vi "main.vi"() -> ()   [LabVIEW 2018]
uses:
  Classes/Main/Status STYP.ctl
  Classes/Video Processor/Video Processor.lvclass
  C:/Users/aaron.jencks/Documents/GitHub/emerson_seed_object_detection/LabVIEW/Projects/Paul's Video Viewer/Classes/Video File/Video File.lvclass
  <vilib>/vision/Image Controls.llb/IMAQ Image.ctl
  <userlib>/Jet Engineering/JET_QSM/Code/Private/JET_QSM_InvalidOption STYP.ctl
  Classes/Video File/Video File.lvclass/Video File.ctl
  <userlib>/Jet Engineering/JET_QSM/Code/Private/JET_QSM - Add State [String API].vi
  3189c987-d43a-4d5a-91ed-d680ee457747.vi
  bcec0ad0-729b-4a4f-bcea-59fd1ae3eb4f.vi
  Classes/Video File/Read Number of Frames.vi
  Classes/Video File/Read Frame Number.vi
  Classes/Standard RMS/Standard RMS.lvclass
  C:/Users/aaron.jencks/Documents/GitHub/emerson_seed_object_detection/LabVIEW/Projects/Paul's Video Viewer/Classes/Standard Averager/Standard Averager.lvclass
  <vilib>/Utility/error.llb/Trim Whitespace.vi
  <vilib>/Utility/error.llb/Error Cluster From Error Code.vi
  Classes/Standard Averager/Standard Averager.lvclass
panel:
  out "Frame Number B":u32
  out "Frame Number A":u32
  in  "Depth Value Boundaries":cluster{dbl, dbl}(slide)={0.0, 7.2727272727272725} scale=0.0..5.0
  in  "Position Boundaries B":cluster{u32, u32}(slide)={0, 99} caption="Playback Boundaries" scale=0.0..298.0
  in  "Position Boundaries A":cluster{u32, u32}(slide)={0, 44} caption="Playback Boundaries" scale=0.0..249.0
  in  "Depth Scale B":dbl caption="Depth Scale"
  in  "Depth Scale A":dbl caption="Depth Scale"
  in  "Averaging Type":enum32{"Normal Average", "RMS"}(radio)
  out "Video B Info":cluster{"Roughness":dbl, "Average Depth":dbl} {"Roughness" format="%#.3g"; "Average Depth" format="%#.3g"}
  out "Video A Info":cluster{"Roughness":dbl, "Average Depth":dbl} {"Roughness" format="%#.3g"; "Average Depth" format="%#.3g"}
  in  "Restart":bool
  in  "stop":bool
  in  "Depth History Length (-1: Infinite)":i32=10
  out "Playback Position":dbl(slide) scale=0.0..100.0
  in  "Pause":bool
  in  "Play":bool
  in  "Video Path B":path
  in  "Video Path A":path
  in  "FPS":dbl(slide) scale=1.0..15.0
  out "Recent states before Error (with tick counts) 2":string="0.167 sec ago: VI Initialize\n0.167 sec ago: Window Open\n0.110 sec ago: Control Update\n0.110 sec ago: Indicator Update\n0.000 sec ago: Error Handler\r\n"
  out "error out":errorcluster
  out "Video Frame B":T1(plugin-control)
  out "Video Frame A":T1(plugin-control)
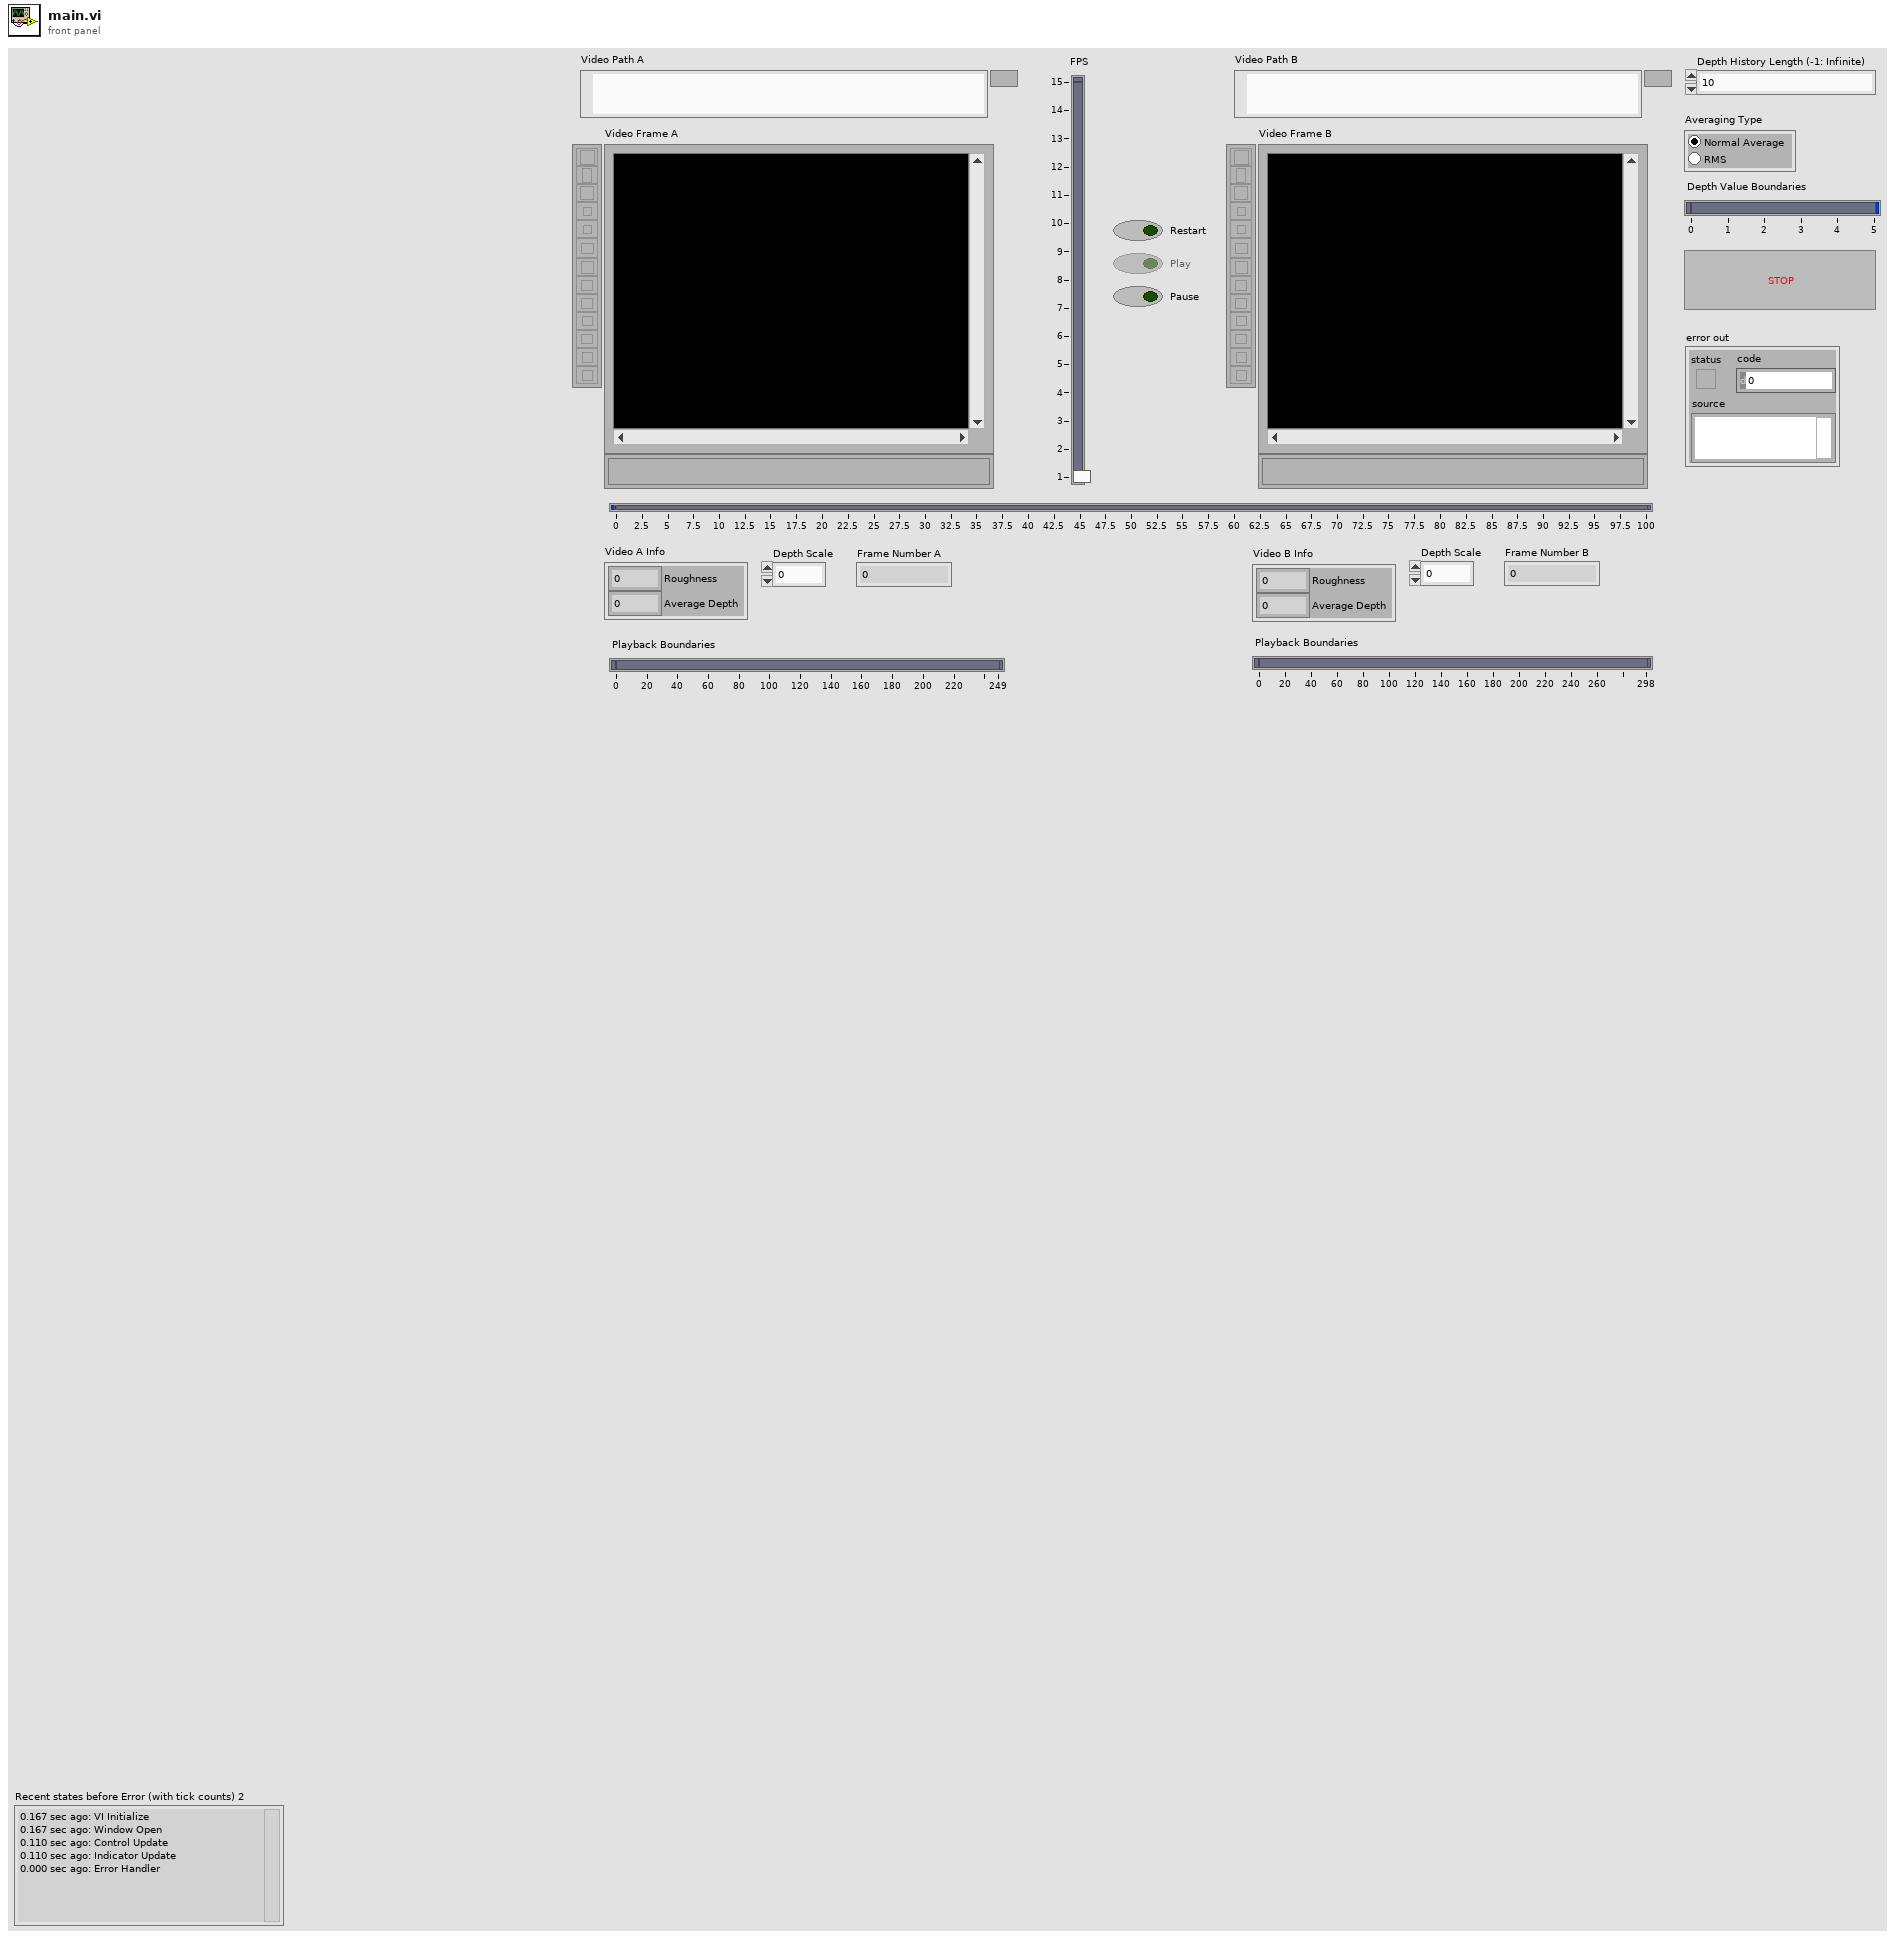
[diagram p1: front panel]
types:
  T1 = typedef "IMAQ Image.ctl" = refnum<image>
  T2 = typedef "Status STYP.ctl" = cluster{"VI":cluster{"error":errorcluster, "isExiting?":bool}, "UserLoggedIn?":bool, "Processors":cluster{"Video A":refnum<class "Video Processor.lvclass">, "Video B":refnum<class "Video Processor.lvclass">, "Averaging Type":enum32{"Normal Average", "RMS"}}, "Playback":cluster{"FPS":dbl, "Playing?":bool, "Playable?":bool, "Image A":T1, "Image B":T1}}
  T3 = typedef "JET_QSM_InvalidOption STYP.ctl" = enum16{"Ignore", "Dialog", "Error"}
  T4 = typedef "JET_QSM_Refnum STYP.ctl" = cluster{"state":cluster{"queue":refnum<queue>, "idle":string, "error":string, "STOP":string}, "debug":cluster{"enabled?":bool, "queue":refnum<queue>}, "Invalid.option":T3, "QSM.Name":string}
  T5 = enum32{"invalid app kind", "Development System", "Run Time System", "Student Edition", "Embedded LabVIEW", "Evaluation", "Custom"}
  T6 = typedef "Image Type" = u32
  T7 = cluster{"Global Rectangle":i32[], "Contours":cluster{"Contour Type":u32, "ROI Type":u32, "Points":i32[]}[]}
  T8 = typedef "JET_QSM_Element STYP.ctl" = cluster{"state":string, "data":variant, "comment":string}
  T9 = cluster{"Number of Frames":u32, "Accessors:Number of Frames":u32}
  T10 = cluster{"Accessors:History Standard Deviation":dbl, "Accessors:History Average":dbl}
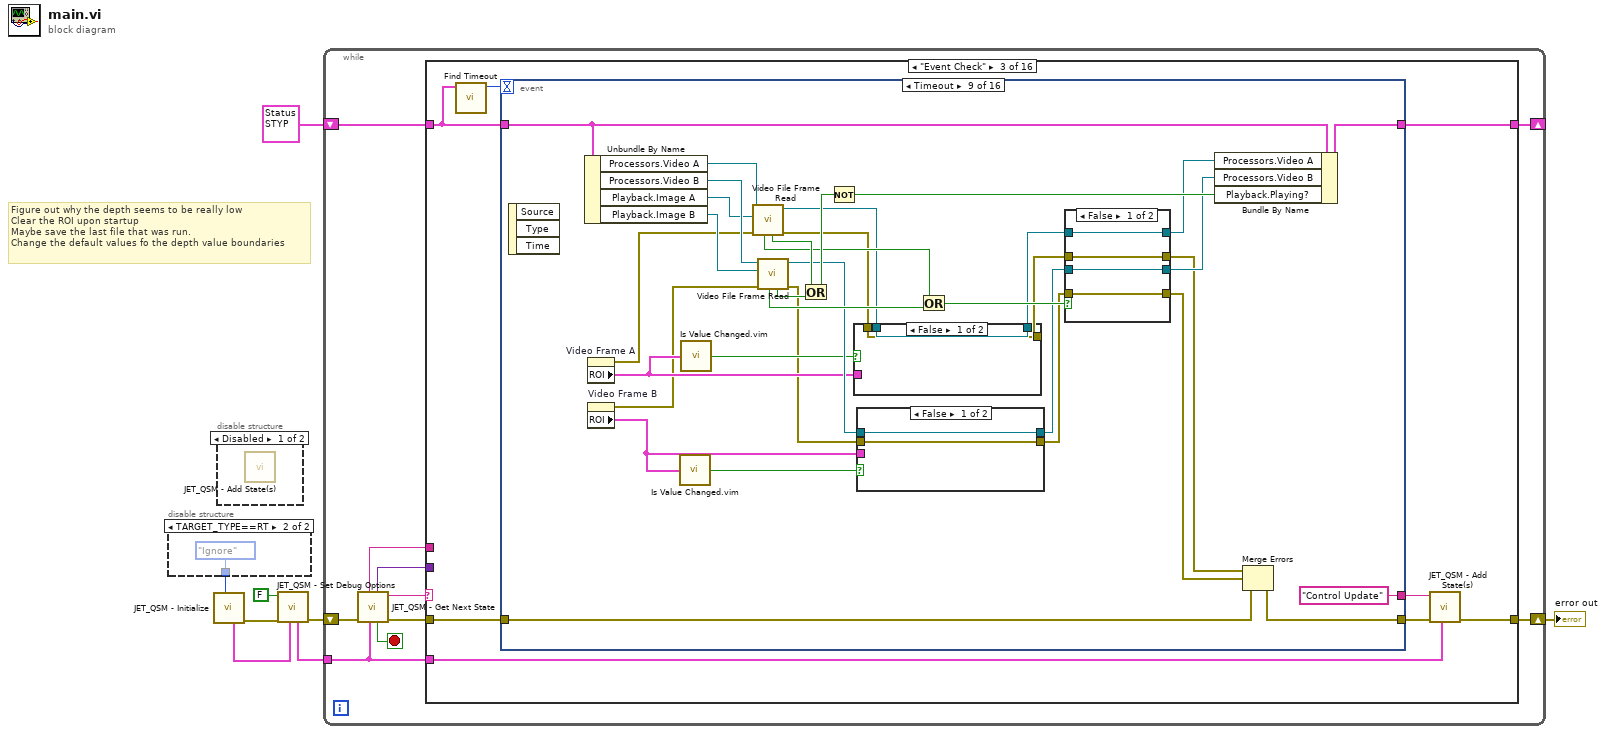
[diagram p0: block diagram]
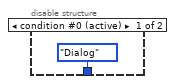
[diagram p2: hidden frame]
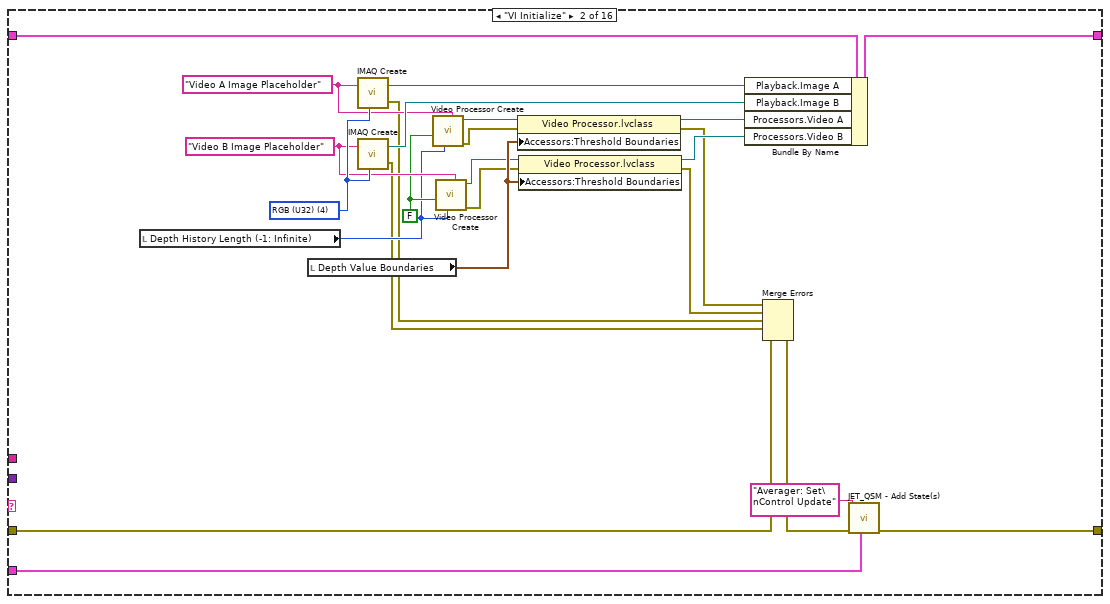
[diagram p5: hidden frame]
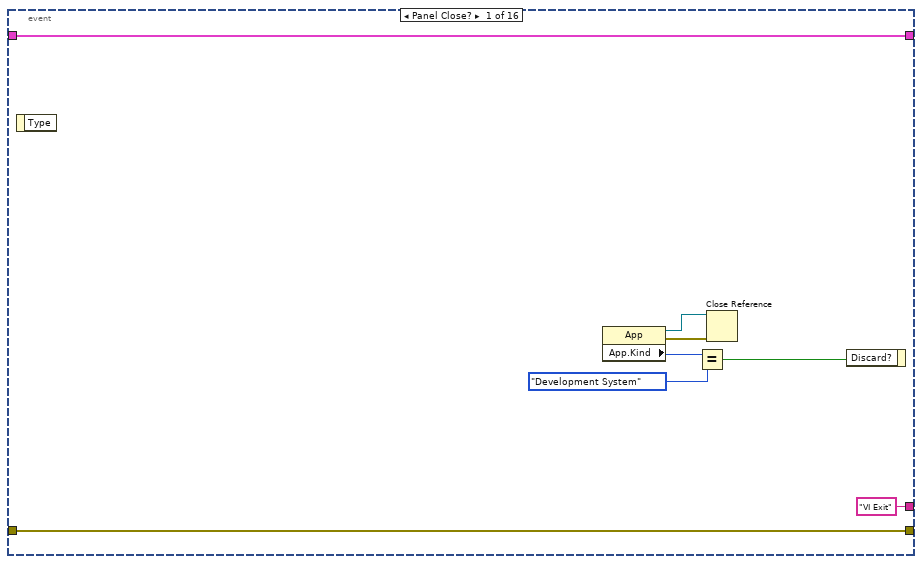
[diagram p6: hidden frame]
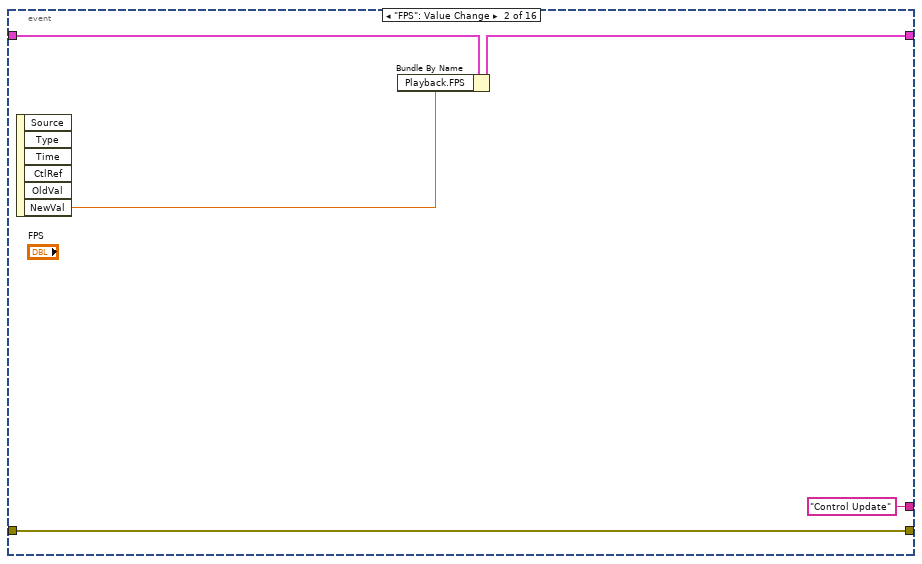
[diagram p7: hidden frame]
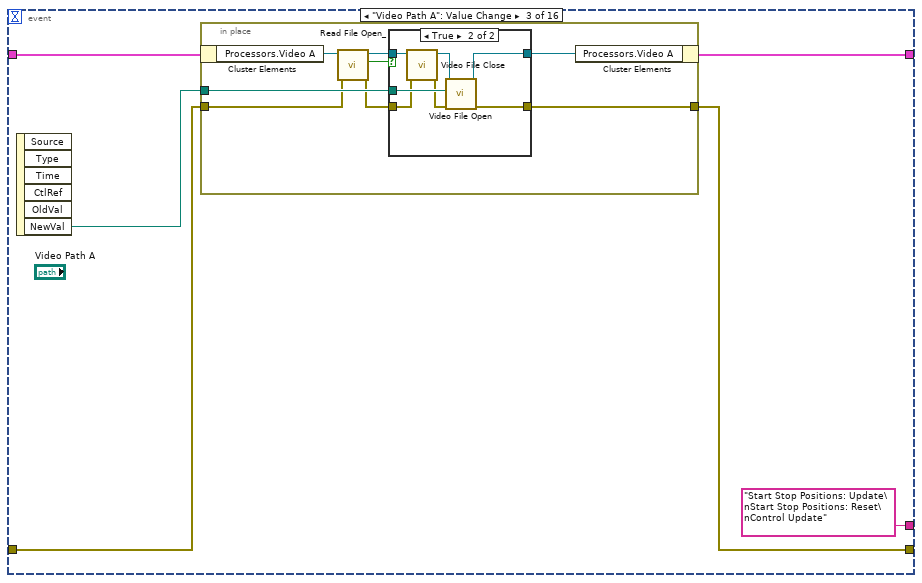
[diagram p8: hidden frame]
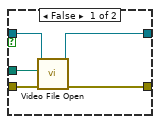
[diagram p9: hidden frame]
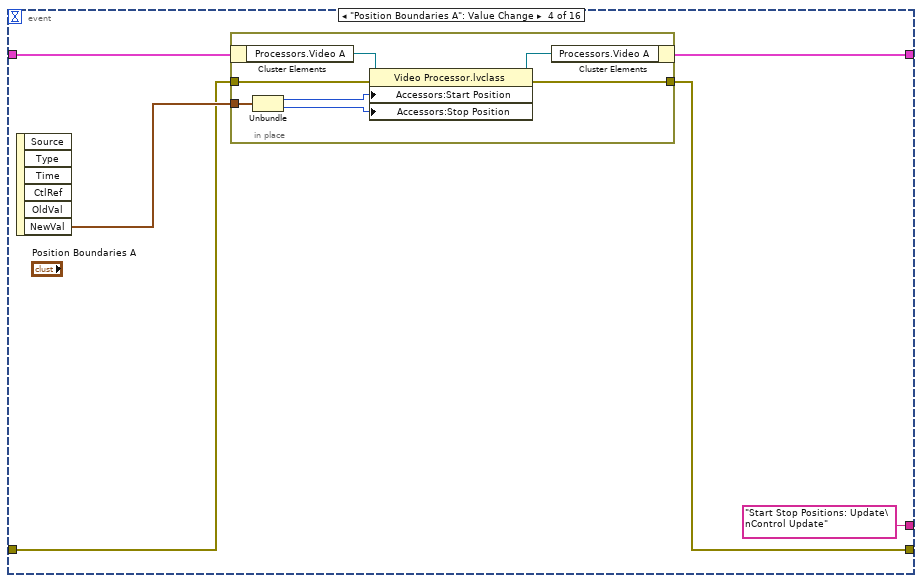
[diagram p10: hidden frame]
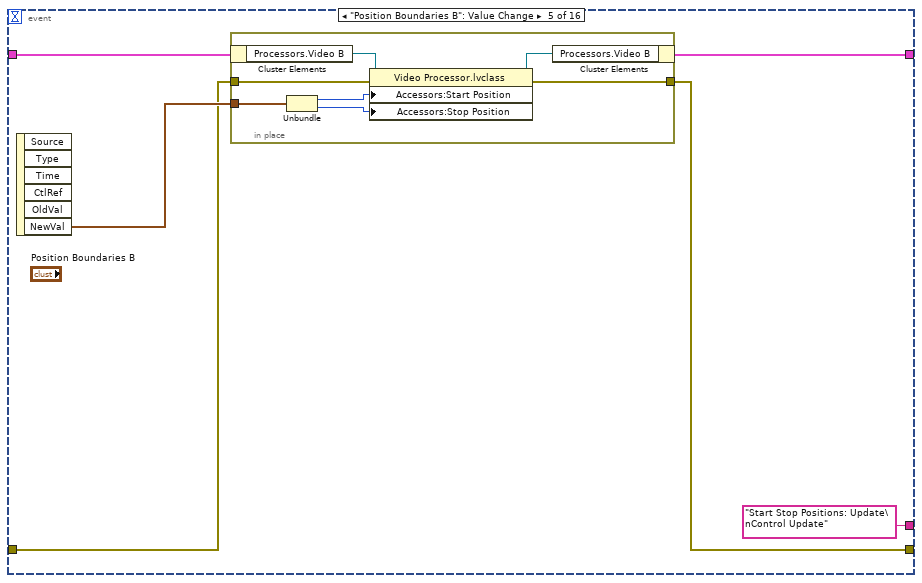
[diagram p11: hidden frame]
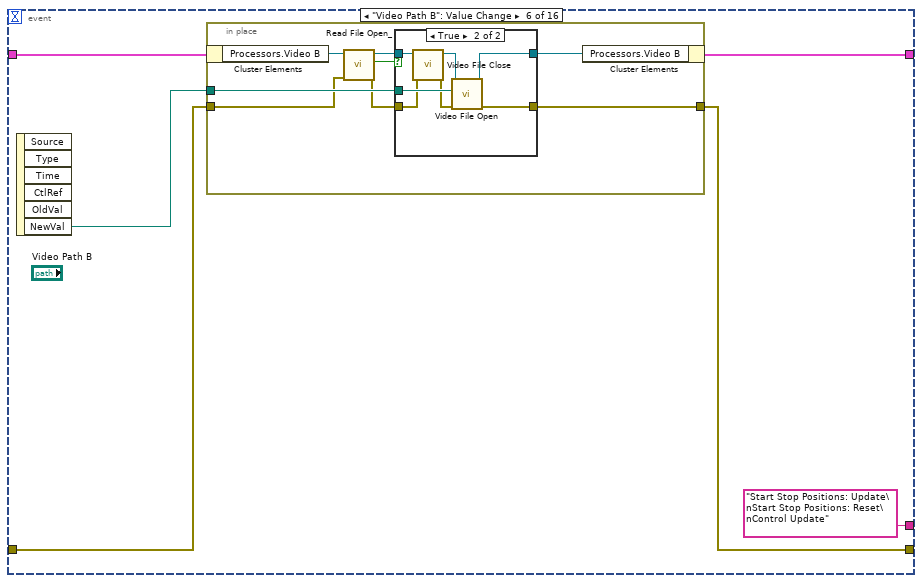
[diagram p12: hidden frame]
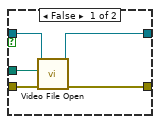
[diagram p13: hidden frame]
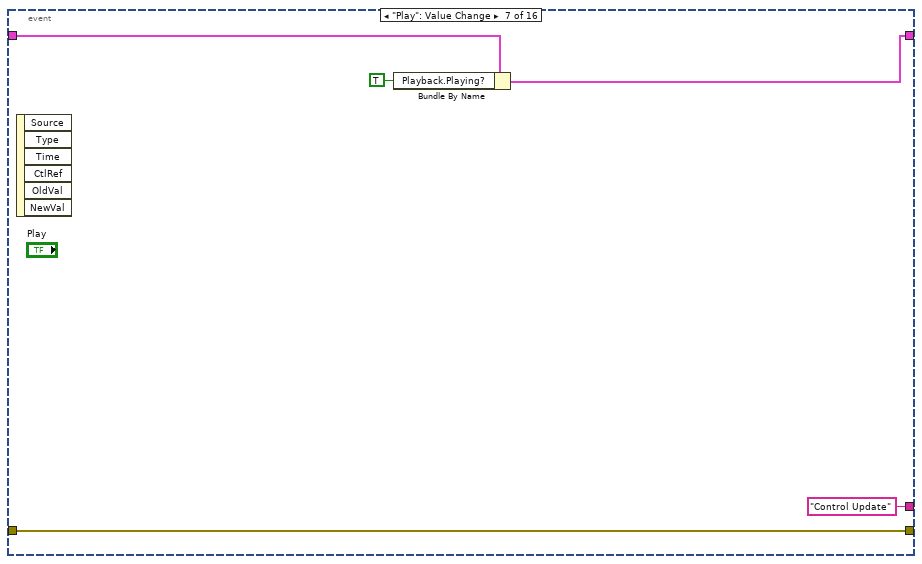
[diagram p14: hidden frame]
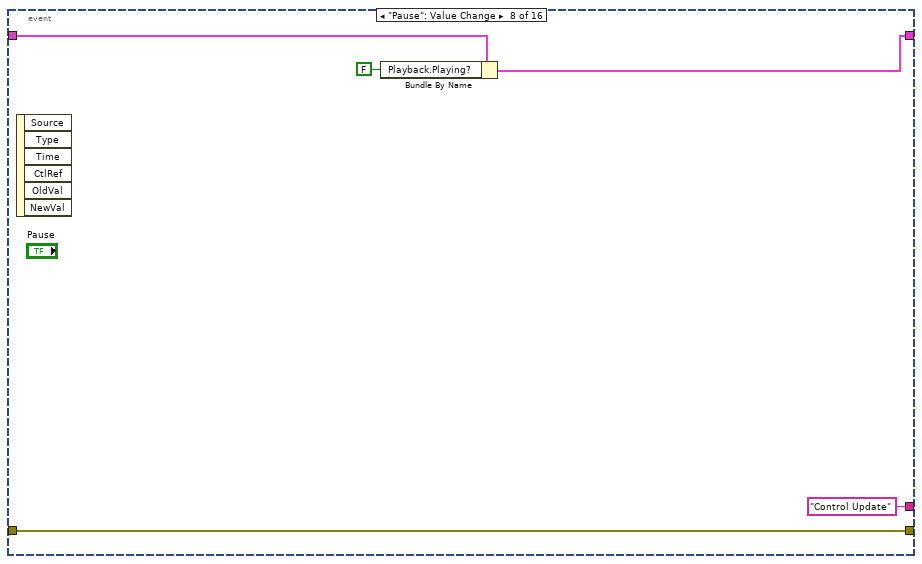
[diagram p15: hidden frame]
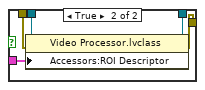
[diagram p16: hidden frame]
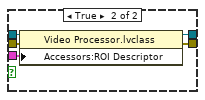
[diagram p17: hidden frame]
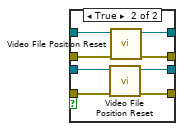
[diagram p18: hidden frame]
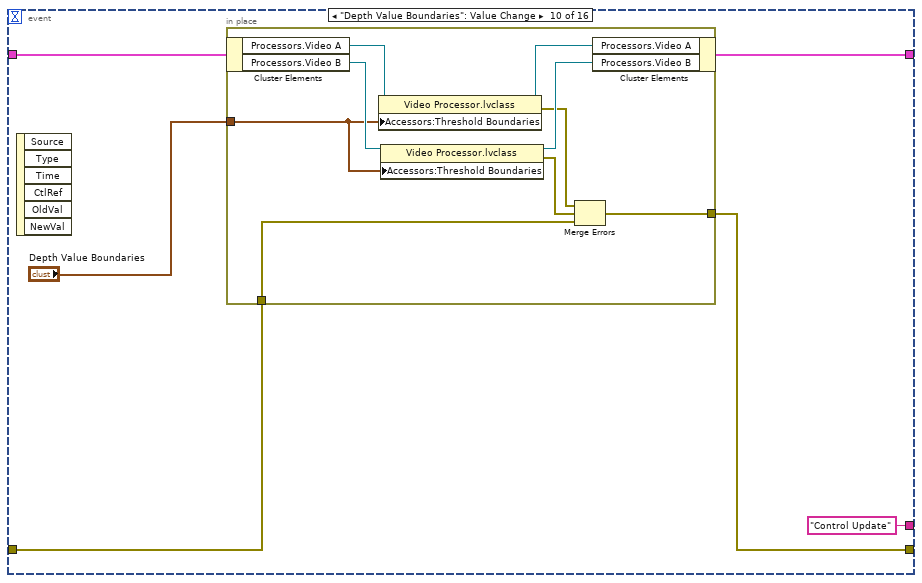
[diagram p19: hidden frame]
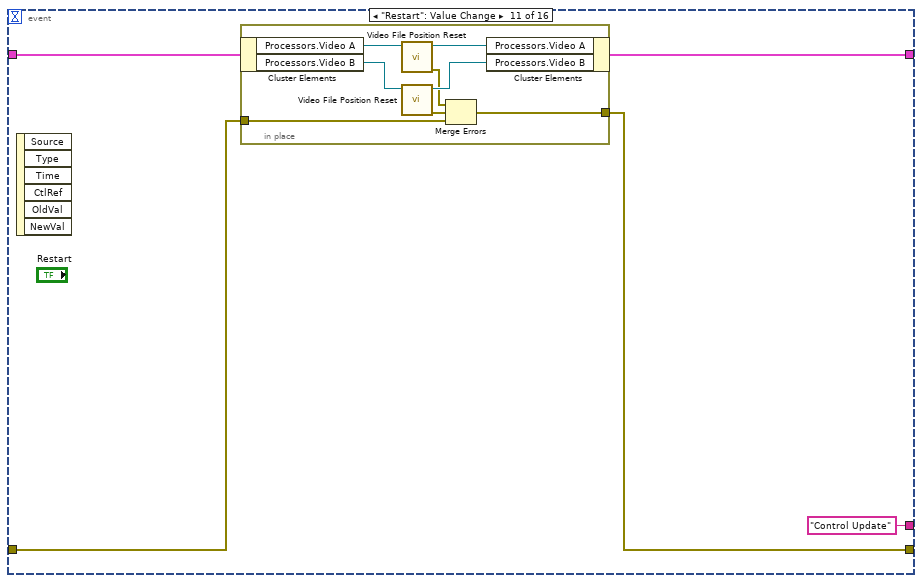
[diagram p20: hidden frame]
diagram:
  # "Figure out why the depth seems to be really low\nClear the ROI upon startup\nMaybe save the last file that was run.\nChange the default values fo the depth value boundaries"
  n1 = disable-structure shown="TARGET_TYPE==RT" {
    disable-tunnel: [JET_QSM_InvalidOption_STYP."Dialog" ("invalid state action (Dialog)") JET_QSM_InvalidOption_STYP."Ignore" ("invalid state action (Dialog)")] -> w8
    frame condition #0 (active) {
    }
    frame condition #1 {
    }
  }
  n2 = call <userlib>:"JET_QSM - Initialize.vi"("invalid state action (Dialog)"=w8) -> ("error out"=w1:errorcluster, "Jet_QSM refnum"=w4:T4)  [unwired: 9 in]
  n3 = disable-structure shown="Disabled" {
    frame Disabled {
      n4 = call-poly <userlib>:"JET_QSM - Add State(s).vi"() -> ()  [unwired: 11 in, 1 out]
    }
    frame Enabled {
    }
  }
  n5 = call <userlib>:"JET_QSM - Set Debug Options.vi"("Jet_QSM refnum"=w4, "error in (no error)"=w1, "debug.enabled? (F)"=FALSE) -> ("error out"=w2:errorcluster, "Jet_QSM ref"=w3:T4)  [unwired: 7 in]
  n6 = while {
    tunnel: w3 -> [w16]
    shift-right: [w14] -> _
    shift-left: T2 {"VI"={"error"={"status"=FALSE, "code"=0, "source"=""}, "isExiting?"=FALSE}, "UserLoggedIn?"=FALSE, "Processors"={"Video A"=refnum, "Video B"=refnum, "Averaging Type"=enum."Normal Average"}, "Playback"={"FPS"=10.0, "Playing?"=FALSE, "Playable?"=FALSE, "Image A"=refnum, "Image B"=refnum}} ("Status") -> [w15]
    shift-right: [w13] -> w7
    shift-left: w2 -> [w20]
    stop <- w17 stop-if-true
    n7 = call <userlib>:"JET_QSM - Get Next State.vi"("Jet_QSM refnum"=w16, "error in (no error)"=w20) -> ("error out"=w19:errorcluster, "state"=w18:string, "Stop Loop?"=w17:bool, "state data"=w12:variant, "state comment"=w11:string)  [unwired: 5 in]
    n8 = case shown="\"Event Check\"" w18 {
      selector: w18 -> [_ _ _ _ _ _ w350 _ _ _ _ _ _ _ _ _]
      tunnel: w19 -> [w21 w23 w55 w311 w342 _ w351 w353 w355 w357 w360 w378 w381 w393 w441 w445]
      tunnel: w16 -> [_ w38 w54 w316 w340 _ w349 _ _ _ _ _ _ _ w442 _]
      tunnel: w15 -> [w22 w47 w49 w312 w338 w346 w352 w354 w356 w358 w363 w379 w391 w405 w434 w462]
      tunnel: [w22 w46 w50 w310 w338 w346 w352 w354 w356 w358 w362 w379 w391 w405 w433 w461] -> w14
      tunnel: [w21 w37 w52 w317 w342 w347 w348 w353 w355 w357 w359 w378 w380 w392 w406 w444] -> w13
      tunnel: w12 -> [_ _ _ _ _ _ _ _ _ _ _ _ _ _ _ _]
      tunnel: w11 -> [_ _ _ _ _ _ _ _ _ _ _ _ _ _ _ _]
      frame "------ Standard States ------" {
        # "Standard States are required states for a JET_QSM State Machine\n\nTheir names may be changed; use the Initialize function to specify the new names"
        # "This is a section header; the state is never expected to execute"
      }
      frame "VI Initialize" {
        w40 = FALSE ("Open File? (T)")
        w42 = "Video B Image Placeholder" ("Image Name")
        w41 = "Video A Image Placeholder" ("Image Name")
        w45 = T6 4 items=["Grayscale (U8)", "Grayscale (I16)", "Grayscale (SGL)", "Complex (CSG)", "RGB (U32)", "HSL (U32)", "RGB (U64)", "Grayscale (U16)"] ("Image Type")
        n9 = local read "Depth History Length (-1: Infinite)"() -> (w39:i32)
        n10 = local read "Depth Value Boundaries"() -> (w35:cluster{dbl, dbl})
        n11 = call "IMAQ Create"("Image Name"=w41, "Image Type"=w45) -> ("New Image"=w44:T1, "error out"=w26:errorcluster)  [unwired: 3 in]
        n12 = call "IMAQ Create"("Image Name"=w42, "Image Type"=w45) -> ("New Image"=w43:T1, "error out"=w25:errorcluster)  [unwired: 3 in]
        n13 = call "Video Processor Create.vi"("Identifier"=w41, "Depth History Size (10)"=w39, "Open File? (T)"=w40) -> ("error out"=w29:errorcluster, "Video Processor out"=w34:refnum<class "Video Processor.lvclass">)  [unwired: 7 in]
        n14 = call "Video Processor Create.vi"("Identifier"=w42, "Depth History Size (10)"=w39, "Open File? (T)"=w40) -> ("error out"=w30:errorcluster, "Video Processor out"=w32:refnum<class "Video Processor.lvclass">)  [unwired: 7 in]
        n15 = property class="Video Processor.lvclass"(reference=w34, error in=w29, "Accessors:Threshold Boundaries"=w35) -> (reference out=w33:refnum<class "Video Processor.lvclass">, error out=w28:errorcluster)
        n16 = property class="Video Processor.lvclass"(reference=w32, error in=w30, "Accessors:Threshold Boundaries"=w35) -> (reference out=w31:refnum<class "Video Processor.lvclass">, error out=w27:errorcluster)
        n17 = Bundle By Name(cluster=w47, "Playback.Image A"=w44, "Playback.Image B"=w43, "Processors.Video A"=w33, "Processors.Video B"=w31) -> (w46:T2)
        n18 = Merge Errors(w28, w27, w26, w25, w23) -> (w24:errorcluster)
        n19 = call-poly <userlib>:"JET_QSM - Add State(s).vi"("Jet_QSM refnum"=w38, "error in (no error)"=w24, "state(s)"="Averager: Set\nControl Update") -> ("error out"=w37:errorcluster)  [unwired: 8 in]
      }
      frame "Event Check" {
        n20 = call "Find Timeout.vi"("Status"=w49) -> ("Timeout"=w48:i32)  [unwired: 10 in]
        n21 = event shown="[8] Timeout" {
          selector: _ -> [_ _ _ _ _ _ _ _ _ _ _ _ _ _ _ _]
          dyn-events: _ -> [_ _ _ _ _ _ _ _ _ _ _ _ _ _ _ _]
          timeout: w48 -> [_ _ _ _ _ _ _ _ _ _ _ _ _ _ _ _]
          tunnel: w55 -> [w57 w68 w71 w96 w109 w125 w151 w156 w157 w218 w233 w249 w251 w262 w272 w288]
          tunnel: ["VI Exit" ("state(s)") "Control Update" ("state(s)") "Start Stop Positions: Update\nStart Stop Positions: Reset\nControl Update" ("state(s)") "Start Stop Positions: Update\nControl Update" ("state(s)") "Start Stop Positions: Update\nControl Update" ("state(s)") "Start Stop Positions: Update\nStart Stop Positions: Reset\nControl Update" ("state(s)") "Control Update" ("state(s)") "Control Update" ("state(s)") "Control Update" ("state(s)") "Control Update" ("state(s)") "Control Update" ("state(s)") "Averager: Set\nControl Update" ("state(s)") "Control Update" ("state(s)") "Control Update" ("state(s)") "Control Update" ("state(s)") "VI Exit" ("state(s)")] -> w53
          tunnel: [w57 w68 w70 w95 w108 w124 w151 w156 w158 w217 w232 _ w250 w261 w274 w287] -> w51
          tunnel: w49 -> [w56 w66 w73 w100 w113 w126 w150 w155 w188 w221 w235 w247 w254 w265 w277 w294]
          tunnel: [w56 w64 w69 w99 w112 w121 w147 w152 w185 w220 w234 w246 w253 w264 w276 w291] -> w50
          tunnel: [_ _ _ _ _ _ _ _ _ _ _ w249 _ _ _ _] -> _
          event Panel Close? {
            n22 = event-data() -> ()  [unwired: 1 in, 1 out]
            n23 = property class="App"() -> (reference out=w59:refnum<vi>, error out=w60:errorcluster, "App.Kind"=w63:T5)  [unwired: 2 in]
            n24 = Equal?(x=w63, y=T5."Development System") -> (x = y?=w61:bool)
            n25 = Close Reference(reference=w59, error in (no error)=w60) -> ()  [unwired: 1 out]
            n26 = event-data("Discard?"=w61) -> ()  [unwired: 1 in, 1 out]
          }
          event "FPS": Value Change {
            n27 = event-data() -> ("NewVal"=w65:dbl)  [unwired: 1 in, 5 out]
            n28 = Bundle By Name(cluster=w66, "Playback.FPS"=w65) -> (w64:T2)
          }
          event "Video Path A": Value Change {
            n29 = event-data() -> ("NewVal"=w72:path)  [unwired: 1 in, 5 out]
            n30 = in-place {
              in-place-border: w72 -> [w82]
              in-place-border: w71 -> [w76]
              in-place-border: [w77] -> w70
              n31 = in-place-cluster #1(w73) -> ("Processors.Video A"=w81:refnum<class "Video Processor.lvclass">)
              n32 = call-dynamic "Read File Open_.vi"("error in (no error)"=w76, "Video File in"=w81) -> ("error out"=w75:errorcluster, "File Open?"=w80:bool, "Video File out"=w79:refnum<class "Video Processor.lvclass">)  [unwired: 7 in]
              n33 = case shown="True" w80 {
                tunnel: w82 -> [w87 w92]
                tunnel: w79 -> [w86 w94]
                tunnel: [w85 w91] -> w78
                tunnel: w75 -> [w84 w88]
                tunnel: [w83 w89] -> w77
                frame False {
                  n34 = call-dynamic "Video File Open.vi"("error in (no error)"=w84, "Path"=w87, "Video File in"=w86) -> ("error out"=w83:errorcluster, "Video File out"=w85:refnum<class "Video Processor.lvclass">)  [unwired: 7 in]
                }
                frame True {
                  n35 = call-dynamic "Video File Close.vi"("error in (no error)"=w88, "Video File in"=w94) -> ("error out"=w90:errorcluster, "Video File out"=w93:refnum<class "Video Processor.lvclass">)  [unwired: 8 in]
                  n36 = call-dynamic "Video File Open.vi"("error in (no error)"=w90, "Path"=w92, "Video File in"=w93) -> ("error out"=w89:errorcluster, "Video File out"=w91:refnum<class "Video Processor.lvclass">)  [unwired: 7 in]
                }
              }
              n37 = in-place-cluster #1("Processors.Video A"=w78) -> (w69:T2)
            }
          }
          event "Position Boundaries A": Value Change {
            n38 = event-data() -> ("NewVal"=w97:cluster{u32, u32})  [unwired: 1 in, 5 out]
            n39 = in-place {
              in-place-border: w97 -> [w105]
              in-place-border: w96 -> [w102]
              in-place-border: [w101] -> w95
              n40 = in-place-cluster #2(w100) -> ("Processors.Video A"=w107:refnum<class "Video Processor.lvclass">)
              n41 = Unbundle(w105) -> (w104:u32, w103:u32)
              n42 = property class="Video Processor.lvclass"(reference=w107, error in=w102, "Accessors:Start Position"=w104, "Accessors:Stop Position"=w103) -> (reference out=w106:refnum<class "Video Processor.lvclass">, error out=w101:errorcluster)
              n43 = in-place-cluster #2("Processors.Video A"=w106) -> (w99:T2)
            }
          }
          event "Position Boundaries B": Value Change {
            n44 = event-data() -> ("NewVal"=w110:cluster{u32, u32})  [unwired: 1 in, 5 out]
            n45 = in-place {
              in-place-border: w110 -> [w118]
              in-place-border: w109 -> [w115]
              in-place-border: [w114] -> w108
              n46 = in-place-cluster #3(w113) -> ("Processors.Video B"=w120:refnum<class "Video Processor.lvclass">)
              n47 = Unbundle(w118) -> (w117:u32, w116:u32)
              n48 = property class="Video Processor.lvclass"(reference=w120, error in=w115, "Accessors:Start Position"=w117, "Accessors:Stop Position"=w116) -> (reference out=w119:refnum<class "Video Processor.lvclass">, error out=w114:errorcluster)
              n49 = in-place-cluster #3("Processors.Video B"=w119) -> (w112:T2)
            }
          }
          event "Video Path B": Value Change {
            n50 = event-data() -> ("NewVal"=w122:path)  [unwired: 1 in, 5 out]
            n51 = in-place {
              in-place-border: w122 -> [w134]
              in-place-border: w125 -> [w128]
              in-place-border: [w129] -> w124
              n52 = in-place-cluster #4(w126) -> ("Processors.Video B"=w133:refnum<class "Video Processor.lvclass">)
              n53 = call-dynamic "Read File Open_.vi"("error in (no error)"=w128, "Video File in"=w133) -> ("error out"=w127:errorcluster, "File Open?"=w132:bool, "Video File out"=w131:refnum<class "Video Processor.lvclass">)  [unwired: 7 in]
              n54 = case shown="True" w132 {
                tunnel: w134 -> [w139 w144]
                tunnel: w131 -> [w138 w146]
                tunnel: [w137 w143] -> w130
                tunnel: w127 -> [w136 w140]
                tunnel: [w135 w141] -> w129
                frame False {
                  n55 = call-dynamic "Video File Open.vi"("error in (no error)"=w136, "Path"=w139, "Video File in"=w138) -> ("error out"=w135:errorcluster, "Video File out"=w137:refnum<class "Video Processor.lvclass">)  [unwired: 7 in]
                }
                frame True {
                  n56 = call-dynamic "Video File Close.vi"("error in (no error)"=w140, "Video File in"=w146) -> ("error out"=w142:errorcluster, "Video File out"=w145:refnum<class "Video Processor.lvclass">)  [unwired: 8 in]
                  n57 = call-dynamic "Video File Open.vi"("error in (no error)"=w142, "Path"=w144, "Video File in"=w145) -> ("error out"=w141:errorcluster, "Video File out"=w143:refnum<class "Video Processor.lvclass">)  [unwired: 7 in]
                }
              }
              n58 = in-place-cluster #4("Processors.Video B"=w130) -> (w121:T2)
            }
          }
          event "Play": Value Change {
            n59 = event-data() -> ()  [unwired: 1 in, 6 out]
            n60 = Bundle By Name(cluster=w150, "Playback.Playing?"=TRUE) -> (w147:T2)
          }
          event "Pause": Value Change {
            n61 = event-data() -> ()  [unwired: 1 in, 6 out]
            n62 = Bundle By Name(cluster=w155, "Playback.Playing?"=FALSE) -> (w152:T2)
          }
          event Timeout {
            n63 = event-data() -> ()  [unwired: 1 in, 3 out]
            n64 = Unbundle By Name(w188) -> ("Processors.Video A"=w190:refnum<class "Video Processor.lvclass">, "Processors.Video B"=w189:refnum<class "Video Processor.lvclass">, "Playback.Image A"=w187:T1, "Playback.Image B"=w186:T1)
            n65 = property on="Video Frame A" class="ImageControl"() -> (error out=w166:errorcluster, "ROI"=w170:T7)  [unwired: 2 in, 1 out]
            n66 = property on="Video Frame B" class="ImageControl"() -> (error out=w165:errorcluster, "ROI"=w169:T7)  [unwired: 2 in, 1 out]
            n67 = call "Is Value Changed.vim"("value"=w169) -> ("changed or first call?"=w168:bool)
            n68 = call "Is Value Changed.vim"("value"=w170) -> ("changed or first call?"=w167:bool)
            n69 = call-dynamic "Video File Frame Read.vi"("error in (no error)"=w166, "Image Dst"=w187, "Video Processor in"=w190) -> ("error out"=w164:errorcluster, "Video Processor out"=w174:refnum<class "Video Processor.lvclass">, "Playback Finished?"=w183:bool, "Looped?"=w178:bool)  [unwired: 4 in, 1 out]
            n70 = call-dynamic "Video File Frame Read.vi"("error in (no error)"=w165, "Image Dst"=w186, "Video Processor in"=w189) -> ("error out"=w163:errorcluster, "Video Processor out"=w173:refnum<class "Video Processor.lvclass">, "Playback Finished?"=w182:bool, "Looped?"=w177:bool)  [unwired: 4 in, 1 out]
            n71 = Or(x=w183, y=w182) -> (x .or. y?=w181:bool)
            n72 = Not(x=w181) -> (.not. x?=w180:bool)
            n73 = case shown="False" w167 {
              tunnel: w174 -> [w192 w197]
              tunnel: [w192 w196] -> w172
              tunnel: w170 -> [_ w195]
              tunnel: w164 -> [w191 w194]
              tunnel: [w191 w193] -> w162
              frame False {
              }
              frame True {
                n74 = property class="Video Processor.lvclass"(reference=w197, error in=w194, "Accessors:ROI Descriptor"=w195) -> (reference out=w196:refnum<class "Video Processor.lvclass">, error out=w193:errorcluster)
              }
            }
            n75 = case shown="False" w168 {
              tunnel: w173 -> [w199 w204]
              tunnel: [w199 w203] -> w171
              tunnel: w169 -> [_ w202]
              tunnel: w163 -> [w198 w201]
              tunnel: [w198 w200] -> w161
              frame False {
              }
              frame True {
                n76 = property class="Video Processor.lvclass"(reference=w204, error in=w201, "Accessors:ROI Descriptor"=w202) -> (reference out=w203:refnum<class "Video Processor.lvclass">, error out=w200:errorcluster)
              }
            }
            n77 = Or(x=w178, y=w177) -> (x .or. y?=w179:bool)
            n78 = case shown="False" w179 {
              tunnel: w172 -> [w208 w216]
              tunnel: w171 -> [w207 w215]
              tunnel: [w208 w214] -> w176
              tunnel: [w207 w213] -> w175
              tunnel: w162 -> [w206 w212]
              tunnel: w161 -> [w205 w211]
              tunnel: [w206 w210] -> w160
              tunnel: [w205 w209] -> w159
              frame False {
              }
              frame True {
                n79 = call-dynamic "Video File Position Reset.vi"("error in (no error)"=w211, "Video File in"=w215) -> ("error out"=w209:errorcluster, "Video File out"=w213:refnum<class "Video Processor.lvclass">)  [unwired: 8 in]
                n80 = call-dynamic "Video File Position Reset.vi"("error in (no error)"=w212, "Video File in"=w216) -> ("error out"=w210:errorcluster, "Video File out"=w214:refnum<class "Video Processor.lvclass">)  [unwired: 8 in]
              }
            }
            n81 = Bundle By Name(cluster=w188, "Processors.Video A"=w176, "Processors.Video B"=w175, "Playback.Playing?"=w180) -> (w185:T2)
            n82 = Merge Errors(w160, w159, w157) -> (w158:errorcluster)
          }
          event "Depth Value Boundaries": Value Change {
            n83 = event-data() -> ()  [unwired: 1 in, 6 out]
            n84 = in-place {
              in-place-border: "Depth Value Boundaries" -> [w227]
              in-place-border: w218 -> [w223]
              in-place-border: [w224] -> w217
              n85 = in-place-cluster #5(w221) -> ("Processors.Video A"=w231:refnum<class "Video Processor.lvclass">, "Processors.Video B"=w230:refnum<class "Video Processor.lvclass">)
              n86 = property class="Video Processor.lvclass"(reference=w231, "Accessors:Threshold Boundaries"=w227) -> (reference out=w229:refnum<class "Video Processor.lvclass">, error out=w226:errorcluster)  [unwired: 1 in]
              n87 = property class="Video Processor.lvclass"(reference=w230, "Accessors:Threshold Boundaries"=w227) -> (reference out=w228:refnum<class "Video Processor.lvclass">, error out=w225:errorcluster)  [unwired: 1 in]
              n88 = Merge Errors(w226, w225, w223) -> (w224:errorcluster)
              n89 = in-place-cluster #5("Processors.Video A"=w229, "Processors.Video B"=w228) -> (w220:T2)
            }
          }
          event "Restart": Value Change {
            n90 = event-data() -> ()  [unwired: 1 in, 6 out]
            n91 = in-place {
              in-place-border: w233 -> [w237]
              in-place-border: [w238] -> w232
              n92 = in-place-cluster #6(w235) -> ("Processors.Video A"=w244:refnum<class "Video Processor.lvclass">, "Processors.Video B"=w242:refnum<class "Video Processor.lvclass">)
              n93 = call-dynamic "Video File Position Reset.vi"("Video File in"=w244) -> ("error out"=w240:errorcluster, "Video File out"=w243:refnum<class "Video Processor.lvclass">)  [unwired: 9 in]
              n94 = call-dynamic "Video File Position Reset.vi"("Video File in"=w242) -> ("error out"=w239:errorcluster, "Video File out"=w241:refnum<class "Video Processor.lvclass">)  [unwired: 9 in]
              n95 = Merge Errors(w240, w239, w237) -> (w238:errorcluster)
              n96 = in-place-cluster #6("Processors.Video A"=w243, "Processors.Video B"=w241) -> (w234:T2)
            }
          }
          event "Averaging Type": Value Change {
            n97 = event-data() -> ("NewVal"=w245:enum32{"Normal Average", "RMS"})  [unwired: 1 in, 5 out]
            n98 = Bundle By Name(cluster=w247, "Processors.Averaging Type"=w245) -> (w246:T2)
          }
          event "Depth Scale A": Value Change {
            n99 = event-data() -> ("NewVal"=w252:dbl)  [unwired: 1 in, 5 out]
            n100 = in-place {
              in-place-border: w252 -> [w258]
              in-place-border: w251 -> [w257]
              in-place-border: [w256] -> w250
              n101 = in-place-cluster #7(w254) -> ("Processors.Video A"=w260:refnum<class "Video Processor.lvclass">)
              n102 = property class="Video Processor.lvclass"(reference=w260, error in=w257, "Accessors:Depth Scale"=w258) -> (reference out=w259:refnum<class "Video Processor.lvclass">, error out=w256:errorcluster)
              n103 = in-place-cluster #7("Processors.Video A"=w259) -> (w253:T2)
            }
          }
          event "Depth Scale B": Value Change {
            n104 = event-data() -> ("NewVal"=w263:dbl)  [unwired: 1 in, 5 out]
            n105 = in-place {
              in-place-border: w263 -> [w269]
              in-place-border: w262 -> [w268]
              in-place-border: [w267] -> w261
              n106 = in-place-cluster #8(w265) -> ("Processors.Video B"=w271:refnum<class "Video Processor.lvclass">)
              n107 = property class="Video Processor.lvclass"(reference=w271, error in=w268, "Accessors:Depth Scale"=w269) -> (reference out=w270:refnum<class "Video Processor.lvclass">, error out=w267:errorcluster)
              n108 = in-place-cluster #8("Processors.Video B"=w270) -> (w264:T2)
            }
          }
          event "Depth History Length (-1: Infinite)": Value Change {
            n109 = event-data() -> ("NewVal"=w275:i32)  [unwired: 1 in, 5 out]
            n110 = in-place {
              in-place-border: w275 -> [w284]
              in-place-border: [w279] -> w274
              in-place-border: w272 -> [w278]
              n111 = in-place-cluster #9(w277) -> ("Processors.Video A"=w286:refnum<class "Video Processor.lvclass">, "Processors.Video B"=w285:refnum<class "Video Processor.lvclass">)
              n112 = property class="Video Processor.lvclass"(reference=w286, "Accessors:Frame History Depth"=w284) -> (reference out=w283:refnum<class "Video Processor.lvclass">, error out=w281:errorcluster)  [unwired: 1 in]
              n113 = property class="Video Processor.lvclass"(reference=w285, "Accessors:Frame History Depth"=w284) -> (reference out=w282:refnum<class "Video Processor.lvclass">, error out=w280:errorcluster)  [unwired: 1 in]
              n114 = Merge Errors(w281, w280, w278) -> (w279:errorcluster)
              n115 = in-place-cluster #9("Processors.Video A"=w283, "Processors.Video B"=w282) -> (w276:T2)
            }
          }
          event "stop": Value Change {
            n116 = event-data() -> ()  [unwired: 1 in, 6 out]
            n117 = Unbundle By Name(w294) -> ("Processors.Video A"=w300:refnum<class "Video Processor.lvclass">, "Processors.Video B"=w299:refnum<class "Video Processor.lvclass">)
            n118 = property class="Video Processor.lvclass"(reference=w299) -> (reference out=w296:refnum<class "Video Processor.lvclass">, "Accessors:File Open_"=w295:bool)  [unwired: 1 in, 1 out]
            n119 = property class="Video Processor.lvclass"(reference=w300) -> (reference out=w297:refnum<class "Video Processor.lvclass">, "Accessors:File Open_"=w298:bool)  [unwired: 1 in, 1 out]
            n120 = case shown="True" w298 {
              tunnel: w297 -> [w306 w309]
              tunnel: [w306 w308] -> w293
              tunnel: [_ w307] -> w290
              frame False {
              }
              frame True {
                n121 = call-dynamic "Video File Close.vi"("Video File in"=w309) -> ("error out"=w307:errorcluster, "Video File out"=w308:refnum<class "Video Processor.lvclass">)  [unwired: 9 in]
              }
            }
            n122 = case shown="True" w295 {
              tunnel: w296 -> [w302 w305]
              tunnel: [w302 w304] -> w292
              tunnel: [_ w303] -> w289
              frame False {
              }
              frame True {
                n123 = call-dynamic "Video File Close.vi"("Video File in"=w305) -> ("error out"=w303:errorcluster, "Video File out"=w304:refnum<class "Video Processor.lvclass">)  [unwired: 9 in]
              }
            }
            n124 = Merge Errors(w290, w289, w288) -> (w287:errorcluster)
            n125 = Bundle By Name(cluster=w294, "Processors.Video A"=w293, "Processors.Video B"=w292) -> (w291:T2)
          }
        }
        n126 = call-poly <userlib>:"JET_QSM - Add State(s).vi"("Jet_QSM refnum"=w54, "error in (no error)"=w51, "state(s)"=w53) -> ("error out"=w52:errorcluster)  [unwired: 8 in]
      }
      frame "Error Handler" {
        # "Add specific error exception handlers here"
        n127 = Get Date/Time In Seconds() -> (seconds since 1Jan1904=w320:timestamp)
        n128 = call <userlib>:"JET_QSM - Flush Debug Queue.vi"("Jet_QSM refnum"=w316) -> ("QSM Elements"=w318:T8[], "Timestamps"=w319:timestamp[])  [unwired: 8 in, 1 out]
        n129 = Bundle By Name(cluster=w312, "VI.error"=w311) -> (w310:T2)
        n130 = Unbundle By Name(w311) -> ("code"=w313:i32)
        n131 = for {
          tunnel: w318 -> [w332] mode=indexing
          tunnel: [w330] -> w322 mode=indexing
          tunnel: w320 -> [w327]
          tunnel: w319 -> [w328] mode=indexing
          n132 = Subtract(x=w327, y=w328) -> (x-y=w326:dbl)
          n133 = To Double Precision Float(number=w326) -> (double precision float=w325:dbl)
          n134 = Unbundle By Name(w332) -> ("state"=w331:string)
          n135 = Format Into String(format string="%.03f sec ago: %s", w325, w331) -> (resulting string=w330:string)  [unwired: 2 in, 1 out]
        }
        n136 = case shown="Default" w313 {
          selector: w313 -> [w334]
          tunnel: [w335] -> w314
          tunnel: w311 -> [w333]
          frame Default {
            w335 = TRUE  # Exit?
            n137 = disable-structure shown="Default" {
              disable-tunnel: w334 -> [w337 _]
              disable-tunnel: w333 -> [w336 _]
              frame condition #0 (active) {
                n138 = call <vilib>:"Simple Error Handler.vi"("error code (no error:0)"=w337, "error in (no error)"=w336) -> ()  [unwired: 3 in, 5 out]
              }
              frame condition #1 {
              }
            }
          }
        }
        n139 = Array To Spreadsheet String(delimiter (Tab)="\n", array=w322, 3:"%s" ("format string")) -> (spreadsheet string=→"Recent states before Error (with tick counts) 2":string)
        n140 = call-poly <userlib>:"JET_QSM - Add State(s).vi"("act? (T)"=w314, "Jet_QSM refnum"=w316, "state(s)"="VI Exit") -> ("error out"=w317:errorcluster)  [unwired: 8 in]
      }
      frame "VI Exit" {
        n141 = flat-sequence {
          tunnel: w342 -> [w345]
          tunnel: [w344] -> w341
          tunnel: w340 -> [w343]
          tunnel: [w343] -> w339
          frame #0 {
            n142 = call <userlib>:"JET_QSM - Flush.vi"("Jet_QSM ref"=w343, "error in (no error)"=w345) -> ("error out"=w344:errorcluster)  [unwired: 8 in, 1 out]
          }
        }
        n143 = call <userlib>:"JET_QSM - Add STOP.vi"("Jet_QSM refnum"=w339, "error in (no error)"=w341) -> ()  [unwired: 9 in, 1 out]
      }
      frame "VI STOP" {
        # "Pass out any error that was cached"
        # "This State is the STOP State.\nIt ALWAYS is the last state to execute."
        n144 = Unbundle By Name(w346) -> ("VI.error"=w347:errorcluster)
      }
      frame "INVALID STATE", Default {
        # "This is the state that handles a state name that is INVALID (there is no state for it in the state machine)"
        n145 = call <userlib>:"JET_QSM - INVALID State.vi"("Jet_QSM refnum"=w349, "error in (no error)"=w351, "state"=w350) -> ("error out"=w348:errorcluster)  [unwired: 8 in]
      }
      frame "------ Menu Commands ------" {
        # "This is a section header; the state is never expected to execute"
      }
      frame "------ Events  ------" {
        # "This is a section header; the state is never expected to execute"
      }
      frame "------ Actions  ------" {
        # "This is a section header; the state is never expected to execute"
      }
      frame "Averager: Set" {
        n146 = in-place {
          in-place-border: [w364] -> w361
          n147 = in-place-cluster #10(w363) -> ("Processors.Video A"=w373:refnum<class "Video Processor.lvclass">, "Processors.Video B"=w372:refnum<class "Video Processor.lvclass">, "Processors.Averaging Type"=w368:enum32{"Normal Average", "RMS"})
          n148 = case shown="\"RMS\"" w368 {
            tunnel: [w375 w377] -> w369
            tunnel: [w374 w376] -> w367
            frame "Normal Average", Default {
              n149 = call "Standard Averager Create.vi"() -> ("error out"=w374:errorcluster, "Standard Averager out"=w375:refnum<class "Standard Averager.lvclass">)  [unwired: 10 in]
            }
            frame "RMS" {
              n150 = call "Standard RMS Create.vi"() -> ("error out"=w376:errorcluster, "Standard RMS out"=w377:refnum<class "Standard RMS.lvclass">)  [unwired: 10 in]
            }
          }
          n151 = property class="Video Processor.lvclass"(reference=w373, error in=w367, "Accessors:Averager"=w369) -> (reference out=w371:refnum<class "Video Processor.lvclass">, error out=w366:errorcluster)
          n152 = property class="Video Processor.lvclass"(reference=w372, error in=w367, "Accessors:Averager"=w369) -> (reference out=w370:refnum<class "Video Processor.lvclass">, error out=w365:errorcluster)
          n153 = in-place-cluster #10("Processors.Video A"=w371, "Processors.Video B"=w370, "Processors.Averaging Type"=w368) -> (w362:T2)
          n154 = Merge Errors(w366, w365) -> (w364:errorcluster)
        }
        n155 = Merge Errors(w361, w360) -> (w359:errorcluster)
      }
      frame "------ Window and Panel Control ------" {
        # "This is a section header; the state is never expected to execute"
      }
      frame "Start Stop Positions: Reset" {
        w386 = u32 0 ("Number of Frames")
        n156 = Unbundle By Name(w391) -> ("Processors.Video A"=w390:refnum<class "Video Processor.lvclass">, "Processors.Video B"=w389:refnum<class "Video Processor.lvclass">)
        n157 = property class="Video Processor.lvclass"(reference=w389) -> (error out=w382:errorcluster, "Accessors:Number of Frames"=w388:u32)  [unwired: 1 in, 1 out]
        n158 = property class="Video Processor.lvclass"(reference=w390) -> (error out=w383:errorcluster, "Accessors:Number of Frames"=w387:u32)  [unwired: 1 in, 1 out]
        n159 = Bundle("Number of Frames"=w386, "Accessors:Number of Frames"=w387) -> (w385:T9)  [unwired: 1 in]
        n160 = Bundle("Number of Frames"=w386, "Accessors:Number of Frames"=w388) -> (w384:T9)  [unwired: 1 in]
        n161 = local write "Position Boundaries A"(w385) -> ()
        n162 = local write "Position Boundaries B"(w384) -> ()
        n163 = Merge Errors(w383, w382, w381) -> (w380:errorcluster)
      }
      frame "Start Stop Positions: Update" {
        w402 = 0.0 ("Scale.Range:Minimum")
        n164 = Unbundle By Name(w405) -> ("Processors.Video A"=w404:refnum<class "Video Processor.lvclass">, "Processors.Video B"=w403:refnum<class "Video Processor.lvclass">)
        n165 = property class="Video Processor.lvclass"(reference=w403) -> (error out=w396:errorcluster, "Accessors:Number of Frames"=w399:u32)  [unwired: 1 in, 1 out]
        n166 = property class="Video Processor.lvclass"(reference=w404) -> (error out=w397:errorcluster, "Accessors:Number of Frames"=w401:u32)  [unwired: 1 in, 1 out]
        n167 = To Double Precision Float(number=w401) -> (double precision float=w400:dbl)
        n168 = To Double Precision Float(number=w399) -> (double precision float=w398:dbl)
        n169 = property on="Position Boundaries B" class="Slide (strict)"(error in=w396, "Scale.Maximum"=w398, "Scale.Minimum"=w402) -> (error out=w394:errorcluster)  [unwired: 1 in, 1 out]
        n170 = property on="Position Boundaries A" class="Slide (strict)"(error in=w397, "Scale.Maximum"=w400, "Scale.Minimum"=w402) -> (error out=w395:errorcluster)  [unwired: 1 in, 1 out]
        n171 = Merge Errors(w395, w394, w393) -> (w392:errorcluster)
      }
      frame "Control Update" {
        # "Update all control properties here from the status cluster\n(Consolidate/reduce property nodes)"
        n172 = call "Determine Playable.vi"("Status"=w434) -> ("Status Out"=w433:T2)  [unwired: 10 in]
        n173 = Unbundle By Name(w433) -> ("Playback.FPS"=w440:dbl, "Processors.Video A"=w439:refnum<class "Video Processor.lvclass">, "Playback.Playing?"=w431:bool, "Playback.Playable?"=w436:bool, "Processors.Video B"=w435:refnum<class "Video Processor.lvclass">, "Processors.Averaging Type"=w427:enum32{"Normal Average", "RMS"})
        n174 = Not(x=w436) -> (.not. x?=w432:bool)
        n175 = Not(x=w431) -> (.not. x?=w430:bool)
        n176 = local write "Averaging Type"(w427) -> ()
        n177 = property class="Video Processor.lvclass"(reference=w439) -> (error out=w413:errorcluster, "Accessors:Frame History Depth"=w438:i32, "Accessors:video path"=w420:path, "Accessors:Depth Scale"=w426:dbl, "Accessors:Threshold Boundaries"=w424:cluster{"Minimum":dbl, "Maximum":dbl})  [unwired: 1 in, 1 out]
        n178 = property class="Video Processor.lvclass"(reference=w435) -> (error out=w414:errorcluster, "Accessors:video path"=w419:path, "Accessors:Depth Scale"=w425:dbl)  [unwired: 1 in, 1 out]
        n179 = And(x=w430, y=w432) -> (x .and. y?=w429:bool)
        n180 = call <userlib>:"VI Control - Disable Control.vi"("Disable? (T)"=w429) -> ("Disabled Attribute"=w428:u8)  [unwired: 7 in, 1 out]
        n181 = call <userlib>:"VI Control - Disable Control.vi"("Disable? (T)"=w432) -> ("Disabled Attribute"=w423:u8)  [unwired: 7 in, 1 out]
        n182 = call <userlib>:"VI Control - Disable Control.vi"("Disable? (T)"=w430) -> ("Disabled Attribute"=w437:u8)  [unwired: 7 in, 1 out]
        n183 = local write "FPS"(w440) -> ()
        n184 = property on="Restart" class="Bool"("DisabledEnum"=w428) -> (error out=w410:errorcluster)  [unwired: 2 in, 1 out]
        n185 = property on="Play" class="Bool"("DisabledEnum"=w423) -> (error out=w409:errorcluster)  [unwired: 2 in, 1 out]
        n186 = property on="Pause" class="Bool"("DisabledEnum"=w437) -> (error out=w408:errorcluster)  [unwired: 2 in, 1 out]
        n187 = call <vilib>:"Is Path and Not Empty.vi"("path"=w420) -> ("Is Path and Not Empty?"=w418:bool)  [unwired: 4 in]
        n188 = call <vilib>:"Is Path and Not Empty.vi"("path"=w419) -> ("Is Path and Not Empty?"=w417:bool)  [unwired: 4 in]
        n189 = local write "Depth History Length (-1: Infinite)"(w438) -> ()
        n190 = local write "Video Path A"(w420) -> ()
        n191 = local write "Depth Scale A"(w426) -> ()
        n192 = local write "Depth Value Boundaries"(w424) -> ()
        n193 = local write "Video Path B"(w419) -> ()
        n194 = local write "Depth Scale B"(w425) -> ()
        n195 = Not(x=w417) -> (.not. x?=w415:bool)
        n196 = Not(x=w418) -> (.not. x?=w416:bool)
        n197 = call <userlib>:"VI Control - Disable Control.vi"("Disable? (T)"=w416) -> ("Disabled Attribute"=w422:u8)  [unwired: 7 in, 1 out]
        n198 = call <userlib>:"VI Control - Disable Control.vi"("Disable? (T)"=w415) -> ("Disabled Attribute"=w421:u8)  [unwired: 7 in, 1 out]
        n199 = property on="Position Boundaries A" class="Slide (strict)"(error in=w414, "DisabledEnum"=w422) -> (error out=w412:errorcluster)  [unwired: 1 in, 1 out]
        n200 = property on="Position Boundaries B" class="Slide (strict)"(error in=w414, "DisabledEnum"=w421) -> (error out=w411:errorcluster)  [unwired: 1 in, 1 out]
        n201 = call-poly <userlib>:"JET_QSM - Add State(s).vi"("Jet_QSM refnum"=w442, "error in (no error)"=w441, "state(s)"="Indicator Update") -> ("error out"=w407:errorcluster)  [unwired: 8 in]
        n202 = Merge Errors(w413, w412, w411, w410, w409, w408, w407) -> (w406:errorcluster)
      }
      frame "Indicator Update" {
        # "Update all indicator values here from the status cluster\n(Eliminate Local Variables)"
        n203 = Unbundle By Name(w462) -> ("Playback.Image A"=→"Video Frame A":T1, "Playback.Image B"=→"Video Frame B":T1, "Processors.Video A"=w457:refnum<class "Video Processor.lvclass">, "Processors.Video B"=w455:refnum<class "Video Processor.lvclass">)
        n204 = property class="Video Processor.lvclass"(reference=w455) -> (error out=w446:errorcluster, "Accessors:History Average"=w450:dbl, "Accessors:History Standard Deviation"=w451:dbl, "Accessors:Frame Number"=→"Frame Number B":u32)  [unwired: 1 in, 1 out]
        n205 = property class="Video Processor.lvclass"(reference=w457) -> (error out=w447:errorcluster, "Accessors:History Average"=w449:dbl, "Accessors:History Standard Deviation"=w448:dbl, "Accessors:Frame Number"=→"Frame Number A":u32)  [unwired: 1 in, 1 out]
        n206 = call "Calculate Playback Position.vi"("Status"=w462) -> ("Position"=→"Playback Position":dbl, "Status Out"=w461:T2)  [unwired: 9 in]
        n207 = Bundle("Accessors:History Standard Deviation"=w451, "Accessors:History Average"=w450) -> (→"Video B Info":T10)  [unwired: 1 in]
        n208 = Bundle("Accessors:History Standard Deviation"=w448, "Accessors:History Average"=w449) -> (→"Video A Info":T10)  [unwired: 1 in]
        n209 = Merge Errors(w447, w446, w445) -> (w444:errorcluster)
      }
    }
  }
  "error out" <- w7
